vi "GetAppMetadataProperty.vi"(8 "No Error":errorcluster, 11 "Name":string(combo)) -> (0 "error out":errorcluster, 3 "Value":string)   [LabVIEW 2024, in "SDL3.lvlib" / "Init.lvlib"]
doc: "<B>Summary</B>\nGet metadata about your app.\n\n<B>Remarks</B>\nThis returns metadata previously set using SDL_SetAppMetadata() or SDL_SetAppMetadataProperty(). See SDL_SetAppMetadataProperty() for the list of available properties and their meanings."
uses:
  Init.lvlib
  Lib/SDL3-32.dll
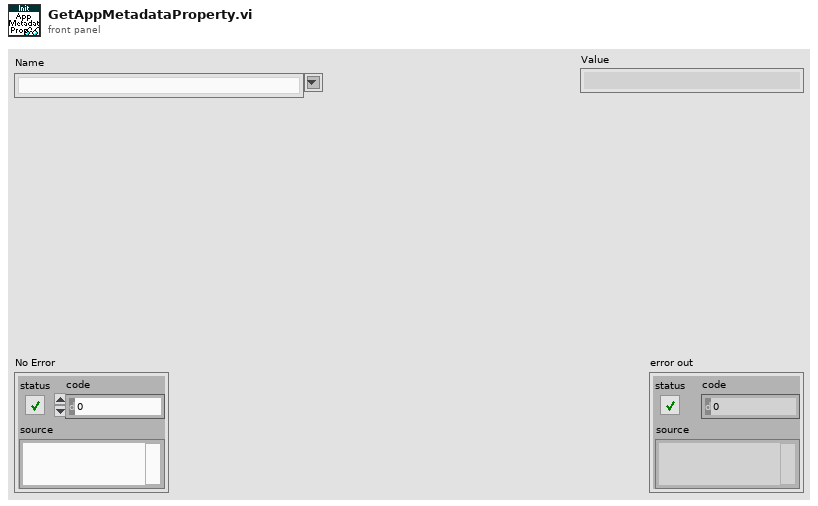
[diagram p1: front panel]
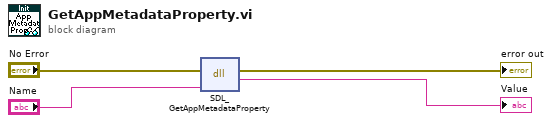
[diagram p0: block diagram]
diagram:
  n1 = dll-call lib="C:/Users/Thomas/Documents/Projects/LV-SDL3/Lib/SDL3-*.*" fn="SDL_GetAppMetadataProperty"(error in="No Error", "name"="Name") -> (error out=→"error out":errorcluster, "return type"=→"Value":string)  [unwired: 3 in, 1 out]
